vi "ReadTDC_link_status.vi"() -> ()   [LabVIEW 2017]
panel:
  out "uart":u8[](array[numeric])
  in  "Port":u16(ring) items=["1", "2", "3", "4", "5", "6", "7", "8", "9", "10", "11", "12"]
  out "Out":u8=94 format="%.0x"
  in  "address":string="192.168.10.35"
  in  "error in (no error)":errorcluster
  out "error out":errorcluster
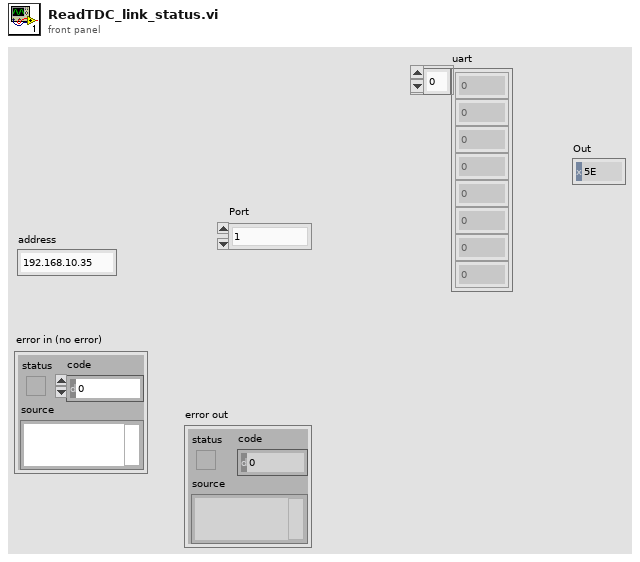
[diagram p1: front panel]
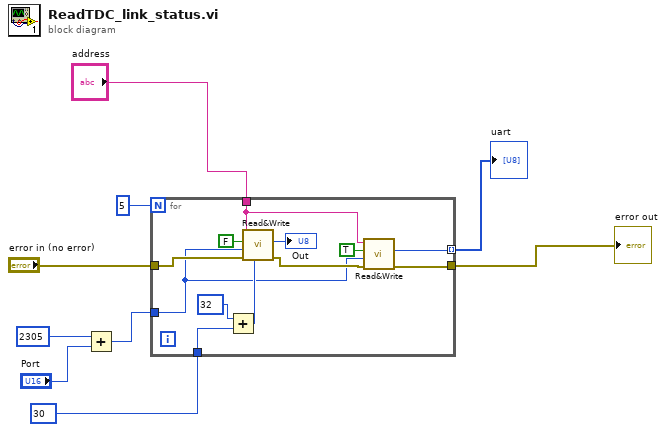
[diagram p0: block diagram]
diagram:
  n1 = Add(x=u32 2305 ("Address"), y="Port") -> (x+y=w1:u32)
  n2 = for {
    N: 5 -> [_]
    tunnel: u8 30 ("In") -> [w18]
    tunnel: "address" -> [w14]
    tunnel: w1 -> [w10]
    tunnel: [w13] -> w4 mode=indexing
    tunnel: "error in (no error)" -> [w20]
    tunnel: [w12] -> w5
    n3 = Add(x=u8 32 ("In"), y=w18) -> (x+y=w17:u8)
    n4 = call "Read&Write.vi"("In"=w17, "error in (no error)"=w20, "Address"=w10, "Read (TRUE)"=FALSE, "address"=w14) -> ("error out"=w11:errorcluster, "Out"=→"Out":u8)  [unwired: 5 in]
    n5 = call "Read&Write.vi"("error in (no error)"=w11, "Address"=w10, "Read (TRUE)"=TRUE, "address"=w14) -> ("error out"=w12:errorcluster, "Out"=w13:u8)  [unwired: 6 in]
  }
  "error out" <- w5
  "uart" <- w4
